vi "Initialize Connection.vi"(8 "error in (no error)":errorcluster, 11 "Sync Box in":refnum<class "Sync Box.lvclass">) -> (0 "error out":errorcluster, 2 "connection ID":refnum<k5>, 3 "Sync Box out":refnum<class "Sync Box.lvclass">)   [LabVIEW 2012, in "Sync Box.lvclass"]
uses:
  Sync Box.lvclass
  Sync Box.lvclass/Sync Box.ctl
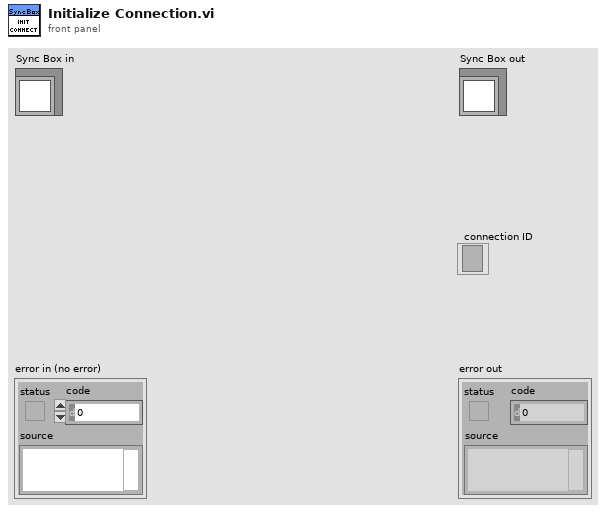
[diagram p1: front panel]
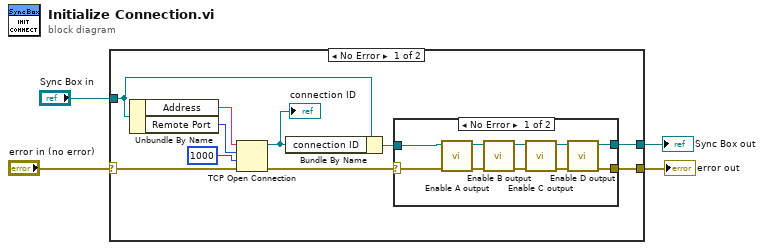
[diagram p0: block diagram]
diagram:
  n1 = case shown="No Error" "error in (no error)" {
    selector: "error in (no error)" -> [w14 w28]
    tunnel: [w7 w28] -> w3
    tunnel: [w5 w27] -> w1
    tunnel: "Sync Box in" -> [w11 w27]
    frame No Error {
      n2 = Unbundle By Name(w11) -> ("Address"=w12:string, "Remote Port"=w13:u32)
      n3 = TCP Open Connection(address=w12, remote port or service name=w13, timeout ms (60000)=1000, error in (no error)=w14) -> (connection ID=w10:refnum<k5>, error out=w8:errorcluster)  [unwired: 1 in]
      "connection ID" <- w10
      n4 = Bundle By Name(cluster=w11, "connection ID"=w10) -> (w6:refnum<class "Sync Box.lvclass">)
      n5 = case shown="No Error" w8 {
        selector: w8 -> [w18 w25]
        tunnel: [w17 w25] -> w7
        tunnel: w6 -> [w16 w26]
        tunnel: [w15 w26] -> w5
        frame No Error {
          n6 = call "Enable A output.vi"("error in (no error)"=w18, "Sync Box in"=w16) -> ("error out"=w24:errorcluster, "Sync Box out"=w19:refnum<class "Sync Box.lvclass">)  [unwired: 8 in]
          n7 = call "Enable B output.vi"("error in (no error)"=w24, "Sync Box in"=w19) -> ("error out"=w23:errorcluster, "Sync Box out"=w20:refnum<class "Sync Box.lvclass">)  [unwired: 8 in]
          n8 = call "Enable C output.vi"("error in (no error)"=w23, "Sync Box in"=w20) -> ("error out"=w22:errorcluster, "Sync Box out"=w21:refnum<class "Sync Box.lvclass">)  [unwired: 8 in]
          n9 = call "Enable D output.vi"("error in (no error)"=w22, "Sync Box in"=w21) -> ("error out"=w17:errorcluster, "Sync Box out"=w15:refnum<class "Sync Box.lvclass">)  [unwired: 8 in]
        }
        frame Error {
        }
      }
    }
    frame Error {
    }
  }
  "error out" <- w3
  "Sync Box out" <- w1
